vi "FaceDL.vi"(0 "Data In":T7 caption="Données en entrée", 2 "Display State In":T5={"Cells_VD2"=enum."5", "position"=0.0, "DS param"={"Domain name"="manip", "experiment"="VD2", "Device Server name"="DLs_VD2", "DL param"={"real pos"=-137.0, "max"=-30.0, "min"=120.0}, "preset pos"=[]}, "event"=refnum} caption="État d'affichage en entrée", 3 "Container State":T6 caption="État du conteneur") -> (6 "Data Out":T7 caption="Données en sortie", 7 "Display State Out":T5={"Cells_VD2"=enum."5", "position"=0.0, "DS param"={"Domain name"="manip", "experiment"="VD2", "Device Server name"="DLs_VD2", "DL param"={"real pos"=-137.0, "max"=-30.0, "min"=120.0}, "preset pos"=[]}, "event"=refnum} caption="État d'affichage en sortie", 8 "Action":T4)   [LabVIEW 2020, in "OWIS_DLs_h.xctl"]
uses:
  OWIS_DLs_h.xctl
  DataDL.ctl
  <vilib>/_xctls/Container State.ctl
  stateDL.ctl
  controls/CellsSDI.ctl
  controls/CellBoolean.ctl
  controls/DLSD.ctl
  <vilib>/_xctls/Action.ctl
  <vilib>/_xctls/XControlSupport.lvlib
panel:
  in  "DS parameters":T1={"Domain name"="manip", "experiment"="VD2", "Device Server name"="DLs_VD2", "DL param"={"real pos"=-137.0, "max"=-30.0, "min"=120.0}, "preset pos"=[-48.0, -24.0, 0.0, 24.0, 48.0]} caption="DeviceServer Param"
  in  "posI":dbl caption="posI,mm"
  in  "DLI":T2=1.0 min=0.0 max=1.0 scale format="%#_6f"
  in  "CellsI":T3
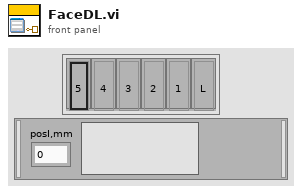
[diagram p1: front panel]
types:
  T1 = cluster{"Domain name":string, "experiment":string, "Device Server name":string, "DL param":cluster{"real pos":dbl, "max":dbl, "min":dbl}, "preset pos":dbl[]}
  T2 = typedef "DLSD.ctl" = dbl
  T3 = typedef "CellsSDI.ctl" = enum32{"5", "4", "3", "2", "1", "L"}
  T4 = typedef "XControlSupport.lvlib/Action.ctl" = cluster{"Data Changed?":bool, "State Changed?":bool, "Action Name":string}
  T5 = typedef "OWIS_DLs_h.xctl/stateDL.ctl" = cluster{"Cells_VD2":T3, "position":dbl, "DS param":cluster{"Domain name":string, "experiment":string, "Device Server name":string, "DL param":cluster{"real pos":dbl, "max":dbl, "min":dbl}, "preset pos":dbl[]}, "event":refnum<user-event>}
  T6 = typedef "XControlSupport.lvlib/Container State.ctl" = cluster{"Indicator?":bool, "Run Mode?":bool, " Refnum":refnum<vi>}
  T7 = typedef "OWIS_DLs_h.xctl/DataDL.ctl" = cluster{"position":dbl}
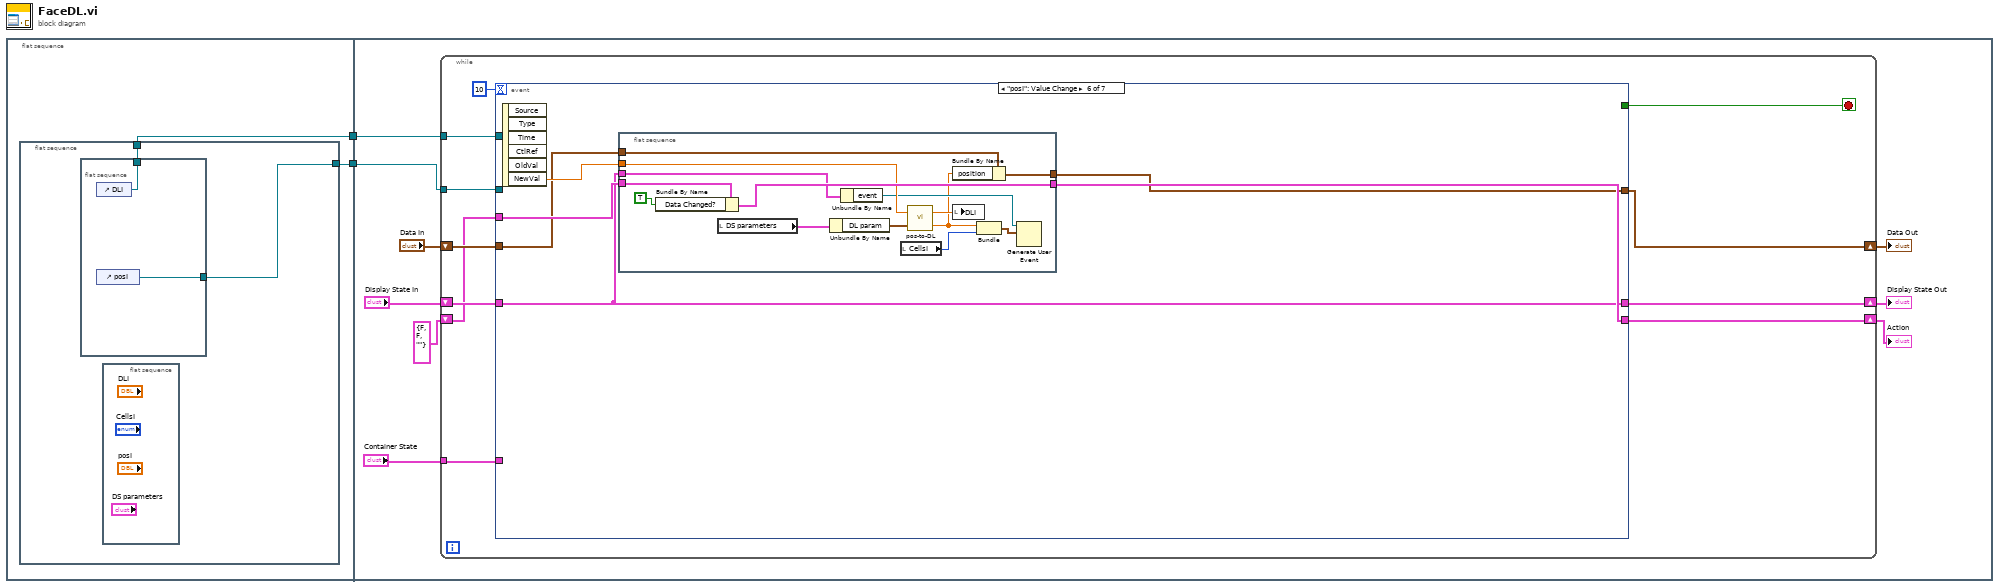
[diagram p0: block diagram]
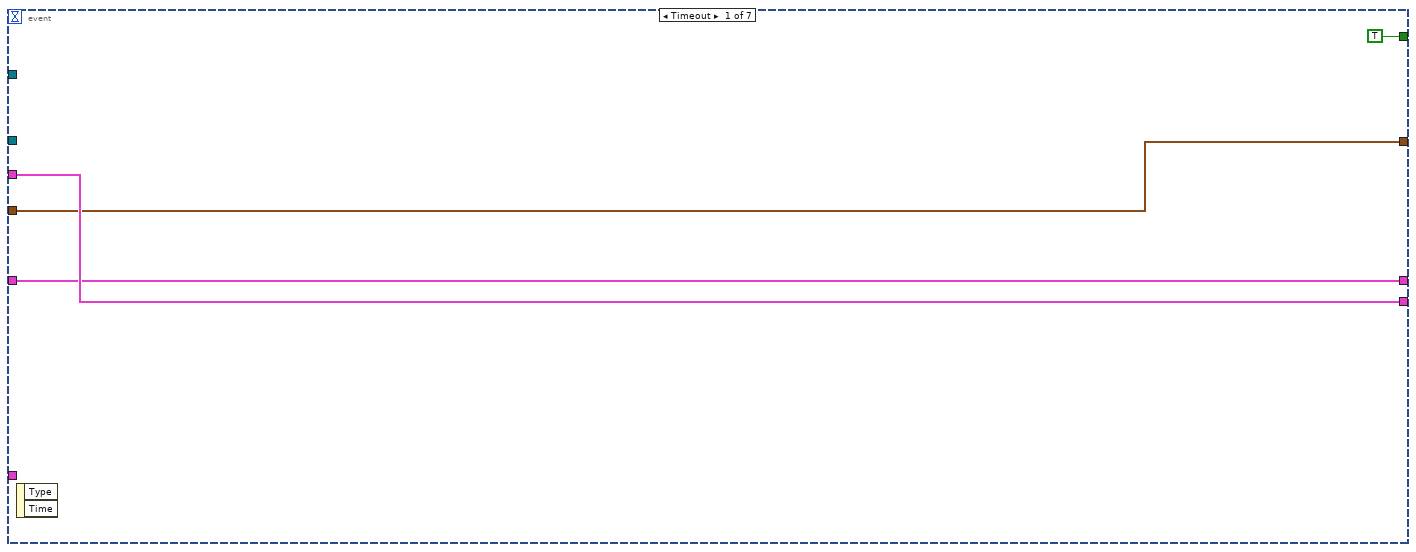
[diagram p2: hidden frame]
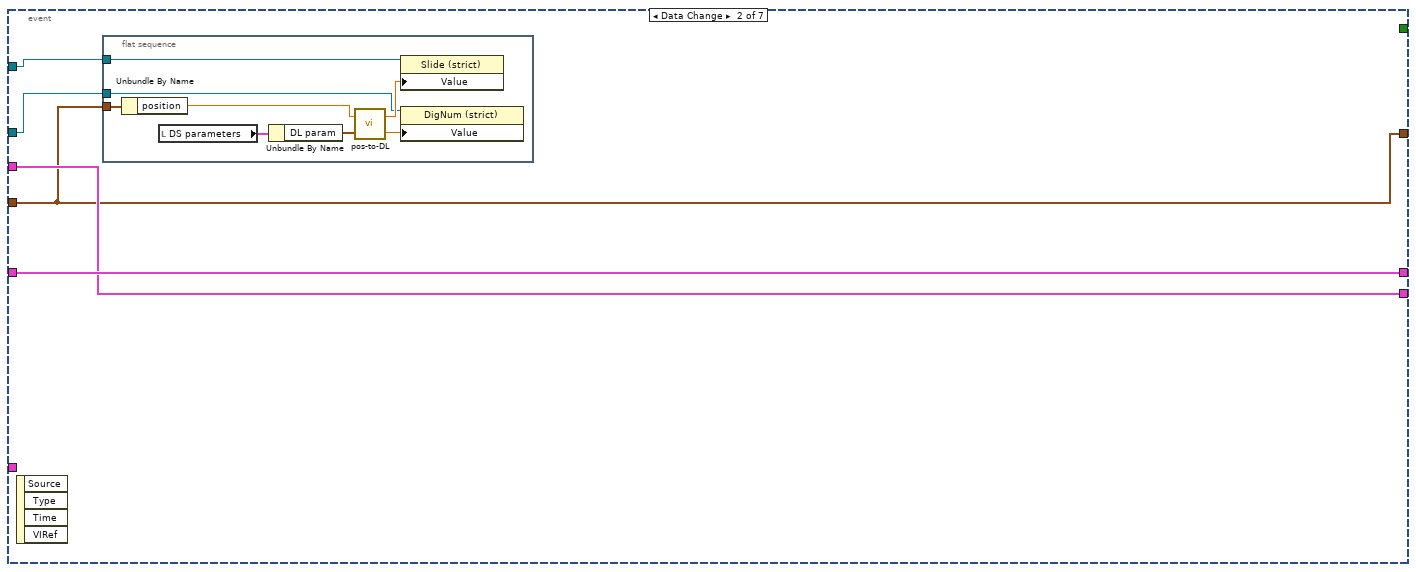
[diagram p3: hidden frame]
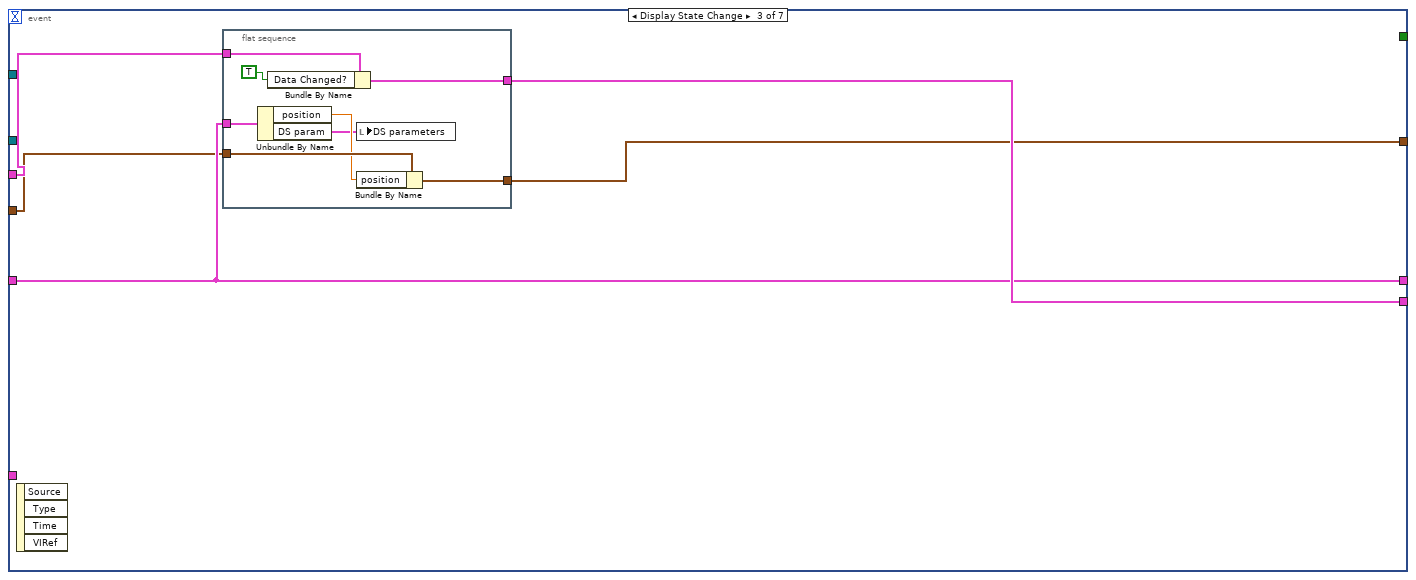
[diagram p4: hidden frame]
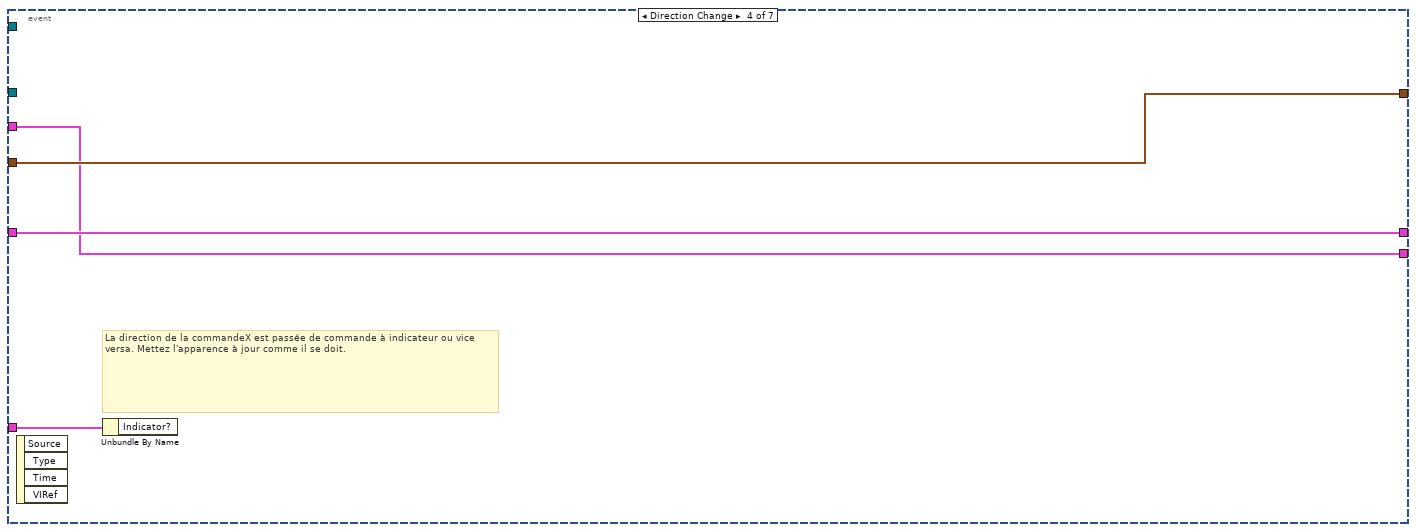
[diagram p5: hidden frame]
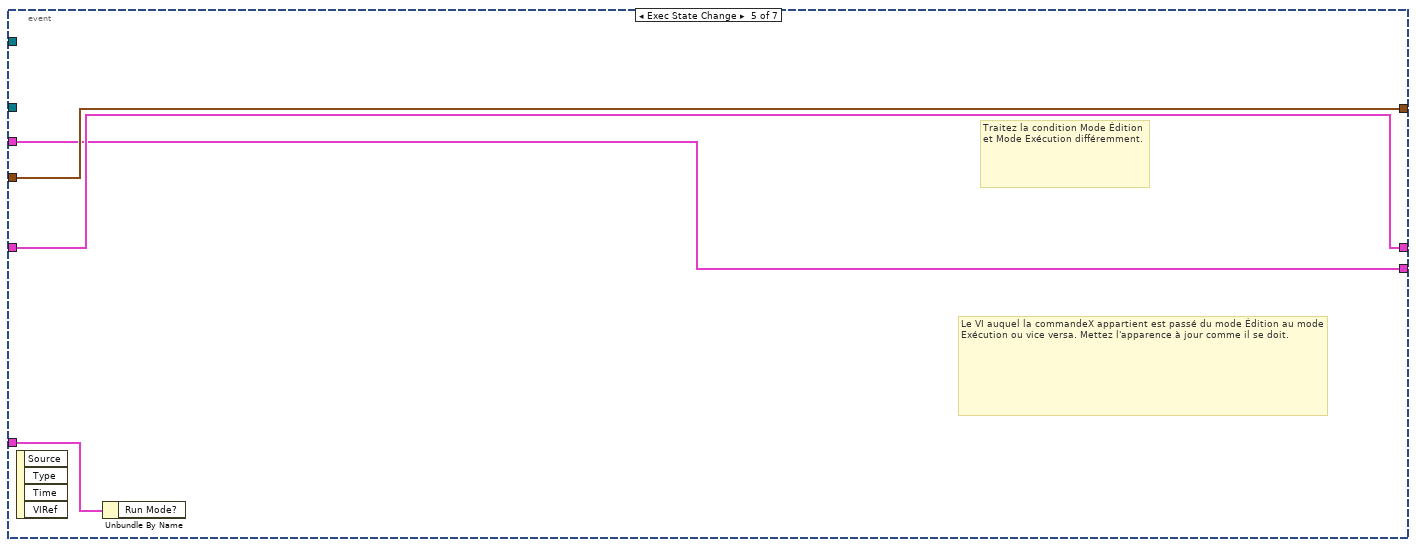
[diagram p6: hidden frame]
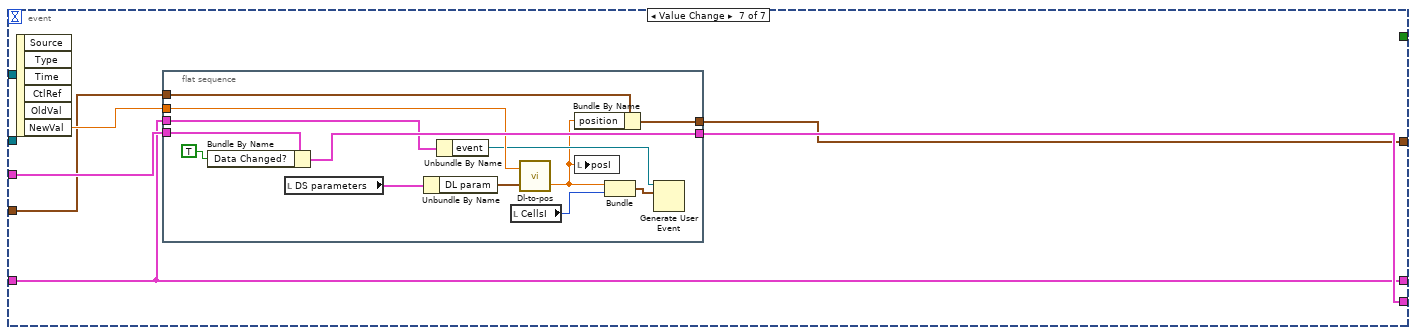
[diagram p7: hidden frame]
diagram:
  n1 = flat-sequence {
    tunnel: [w4] -> w2
    tunnel: [w3] -> w1
    tunnel: w2 -> [w10]
    tunnel: w1 -> [w9]
    frame #0 {
      n2 = flat-sequence {
        tunnel: [w6] -> w4
        tunnel: [w5] -> w3
        frame #0 {
          n3 = flat-sequence {
            tunnel: [w8] -> w6
            tunnel: [w7] -> w5
            frame #0 {
              n4 = control-ref of="DLI"() -> (w8:refnum<vi>)
              n5 = control-ref of="posI"() -> (w7:refnum<vi>)
            }
          }
          n6 = flat-sequence {
            frame #0 {
            }
          }
        }
      }
    }
    frame #1 {
      n7 = while {
        shift-right: [w27] -> w14
        shift-left: "Display State In" -> [w28]
        tunnel: "Container State" -> [w24]
        shift-right: [w22] -> w17
        shift-left: "Data In" -> [w23]
        shift-right: [w20] -> w13
        shift-left: T4 {"Data Changed?"=FALSE, "State Changed?"=FALSE, "Action Name"=""} ("Action") -> [w21]
        tunnel: w10 -> [w19]
        tunnel: w9 -> [w18]
        stop <- w26 stop-if-true
        n8 = event shown="[5] \"posI\": Value Change" {
          selector: _ -> [_ _ _ _ _ _ _]
          dyn-events: _ -> [_ _ _ _ _ _ _]
          timeout: 10 -> [_ _ _ _ _ _ _]
          tunnel: w28 -> [w30 w37 w48 w61 w65 w68 w88]
          tunnel: [w30 w37 w48 w61 w65 w68 w88] -> w27
          tunnel: [TRUE _ _ _ _ _ _] -> w26
          tunnel: w24 -> [_ _ _ w62 w66 _ _]
          tunnel: w23 -> [w29 w35 w47 w60 w64 w67 w87]
          tunnel: [w29 w35 w46 w60 w64 w70 w90] -> w22
          tunnel: [w31 w36 w49 w59 w63 w71 w91] -> w20
          tunnel: w21 -> [w31 w36 w50 w59 w63 w72 w92]
          tunnel: w19 -> [_ w34 _ _ _ _ _]
          tunnel: w18 -> [_ w33 _ _ _ _ _]
          event Timeout {
            n9 = event-data() -> ()  [unwired: 1 in, 2 out]
          }
          event Data Change {
            n10 = event-data() -> ()  [unwired: 1 in, 4 out]
            n11 = flat-sequence {
              tunnel: w35 -> [w45]
              tunnel: w34 -> [w41]
              tunnel: w33 -> [w40]
              frame #0 {
                n12 = Unbundle By Name(w45) -> ("position"=w44:dbl)
                n13 = local read "DS parameters"() -> (w39:T1)
                n14 = Unbundle By Name(w39) -> ("DL param"=w38:cluster{"real pos":dbl, "max":dbl, "min":dbl})
                n15 = call "pos-to-DL.vi"("DL param"=w38, "pos, mm"=w44) -> ("pos, mm"=w43:dbl, "DL pos"=w42:dbl)
                n16 = property class="Slide (strict)"(reference=w41, "Value"=w42) -> ()  [unwired: 1 in, 2 out]
                n17 = property class="DigNum (strict)"(reference=w40, "Value"=w43) -> ()  [unwired: 1 in, 2 out]
              }
            }
          }
          event Display State Change {
            n18 = event-data() -> ()  [unwired: 1 in, 4 out]
            n19 = flat-sequence {
              tunnel: w50 -> [w58]
              tunnel: [w57] -> w49
              tunnel: w48 -> [w55]
              tunnel: w47 -> [w54]
              tunnel: [w53] -> w46
              frame #0 {
                n20 = Unbundle By Name(w55) -> ("position"=w52:dbl, "DS param"=w51:T1)
                n21 = Bundle By Name(cluster=w58, "Data Changed?"=TRUE) -> (w57:T4)
                n22 = local write "DS parameters"(w51) -> ()
                n23 = Bundle By Name(cluster=w54, "position"=w52) -> (w53:T7)
              }
            }
          }
          event Direction Change {
            # "La direction de la commandeX est passée de commande à indicateur ou vice versa. Mettez l'apparence à jour comme il se doit."
            n24 = event-data() -> ()  [unwired: 1 in, 4 out]
            n25 = Unbundle By Name(w62) -> ()  [unwired: 1 out]
          }
          event Exec State Change {
            # "Le VI auquel la commandeX appartient est passé du mode Édition au mode Exécution ou vice versa. Mettez l'apparence à jour comme il se doit."
            # "Traitez la condition Mode Édition et Mode Exécution différemment."
            n26 = event-data() -> ()  [unwired: 1 in, 4 out]
            n27 = Unbundle By Name(w66) -> ()  [unwired: 1 out]
          }
          event "posI": Value Change {
            n28 = event-data() -> ("NewVal"=w69:dbl)  [unwired: 1 in, 5 out]
            n29 = flat-sequence {
              tunnel: w72 -> [w86]
              tunnel: [w85] -> w71
              tunnel: [w83] -> w70
              tunnel: w69 -> [w82]
              tunnel: w68 -> [w81]
              tunnel: w67 -> [w80]
              frame #0 {
                n30 = Bundle By Name(cluster=w86, "Data Changed?"=TRUE ("State Changed?")) -> (w85:T4)
                n31 = local read "DS parameters"() -> (w76:T1)
                n32 = Unbundle By Name(w76) -> ("DL param"=w75:cluster{"real pos":dbl, "max":dbl, "min":dbl})
                n33 = Unbundle By Name(w81) -> ("event"=w78:refnum<user-event>)
                n34 = local read "CellsI"() -> (w79:T3)
                n35 = call "pos-to-DL.vi"("DL param"=w75, "pos, mm"=w82) -> ("pos, mm"=w74:dbl, "DL pos"=w77:dbl)
                n36 = Bundle By Name(cluster=w80, "position"=w74) -> (w83:T7)
                n37 = local write "DLI"(w77) -> ()
                n38 = Bundle("pos, mm"=w74, "CellsI"=w79) -> (w73:cluster{"pos, mm":dbl, "CellsI":T3})  [unwired: 1 in]
                n39 = Generate User Event(user event=w78, event data cluster=w73) -> ()  [unwired: 2 in, 2 out]
              }
            }
          }
          event Value Change {
            n40 = event-data() -> ("NewVal"=w89:T2)  [unwired: 1 in, 5 out]
            n41 = flat-sequence {
              tunnel: w92 -> [w105]
              tunnel: [w104] -> w91
              tunnel: [w102] -> w90
              tunnel: w89 -> [w98]
              tunnel: w88 -> [w101]
              tunnel: w87 -> [w100]
              frame #0 {
                n42 = Bundle By Name(cluster=w105, "Data Changed?"=TRUE ("State Changed?")) -> (w104:T4)
                n43 = local read "DS parameters"() -> (w95:T1)
                n44 = Unbundle By Name(w95) -> ("DL param"=w94:cluster{"real pos":dbl, "max":dbl, "min":dbl})
                n45 = Unbundle By Name(w101) -> ("event"=w97:refnum<user-event>)
                n46 = local read "CellsI"() -> (w99:T3)
                n47 = call "Dl-to-pos.vi"("DL param"=w94, "DL_pos"=w98) -> ("pos, mm"=w96:dbl)  [unwired: 1 out]
                n48 = Bundle By Name(cluster=w100, "position"=w96) -> (w102:T7)
                n49 = local write "posI"(w96) -> ()
                n50 = Bundle("pos, mm"=w96, "CellsI"=w99) -> (w93:cluster{"pos, mm":dbl, "CellsI":T3})  [unwired: 1 in]
                n51 = Generate User Event(user event=w97, event data cluster=w93) -> ()  [unwired: 2 in, 2 out]
              }
            }
          }
        }
      }
      "Display State Out" <- w14
      "Data Out" <- w17
      "Action" <- w13
    }
  }
